vi "StartTrial.vi"(8 "error in (no error)":errorcluster, 11 "TrialBasedExperiment in":refnum<class "BehaviorClassification.lvclass">) -> (0 "error out":errorcluster, 3 "TrialBasedExperiment out":refnum<class "BehaviorClassification.lvclass">)   [LabVIEW 2010, in "BehaviorClassification.lvclass"]
uses:
  BehaviorClassification.lvclass
  MatlabExperiment/MatlabExperiment.lvclass
  Matlab API/Matlab API.lvlib
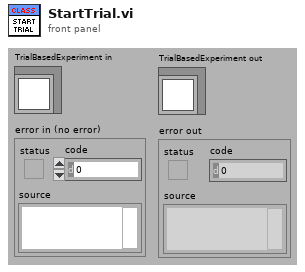
[diagram p1: front panel]
types:
  T1 = cluster{"Intertrial":dbl, "AcquireFixation":dbl, "HoldFixation":dbl, "DelayPeriod":dbl, "ResponsePeriod":dbl}
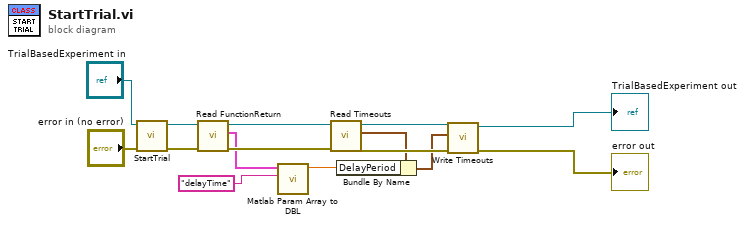
[diagram p0: block diagram]
diagram:
  n1 = call-parent "StartTrial.vi"("error in (no error)"="error in (no error)", "TrialBasedExperiment in"="TrialBasedExperiment in") -> ("error out"=w12:errorcluster, "TrialBasedExperiment out"=w13:refnum<class "BehaviorClassification.lvclass">)  [unwired: 8 in]
  n2 = call-dynamic "Read FunctionReturn.vi"("error in (no error)"=w12, "MatlabExperiment in"=w13) -> ("error out"=w5:errorcluster, "FunctionReturn"=w4:cluster{"Name":string, "Data":variant}[], "MatlabExperiment out"=w10:refnum<class "BehaviorClassification.lvclass">)  [unwired: 7 in]
  n3 = call "Matlab Param Array to DBL.vi"("Name"="delayTime", "Matlab Param Array"=w4) -> ("data"=w2:dbl)  [unwired: 8 in, 1 out]
  n4 = call-dynamic "Read Timeouts.vi"("error in (no error)"=w5, "TrialBasedExperiment in"=w10) -> ("error out"=w6:errorcluster, "Timeouts"=w3:T1, "TrialBasedExperiment out"=w9:refnum<class "BehaviorClassification.lvclass">)  [unwired: 7 in]
  n5 = Bundle By Name(cluster=w3, "DelayPeriod"=w2) -> (w1:T1)
  n6 = call-dynamic "Write Timeouts.vi"("error in (no error)"=w6, "Timeouts"=w1, "TrialBasedExperiment in"=w9) -> ("error out"=→"error out":errorcluster, "TrialBasedExperiment out"=→"TrialBasedExperiment out":refnum<class "BehaviorClassification.lvclass">)  [unwired: 7 in]
